vi "Check PC Time.vi"(8 "Error in":errorcluster, 11 "License File Data Out":T1) -> (0 "Error out":errorcluster, 3 "ValidTime?":bool)   [LabVIEW 2022 SP3]
uses:
  Controls/License Types.ctl
  Controls/License File Data.ctl
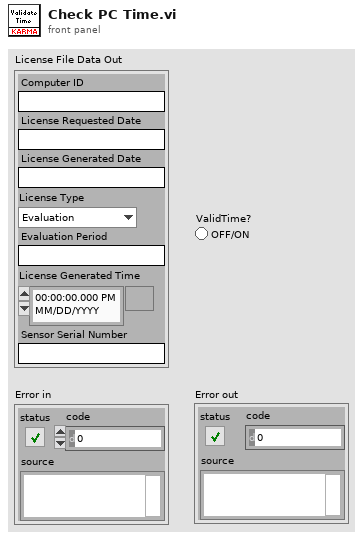
[diagram p1: front panel]
types:
  T1 = typedef "License File Data.ctl" = cluster{"Computer ID":string, "License Requested Date":string, "License Generated Date":string, "License Type":T2, "Evaluation Period":string, "License Generated Time":timestamp, "Sensor Serial Number":string}
  T2 = typedef "License Types.ctl" = enum16{"Evaluation", "Professional"}
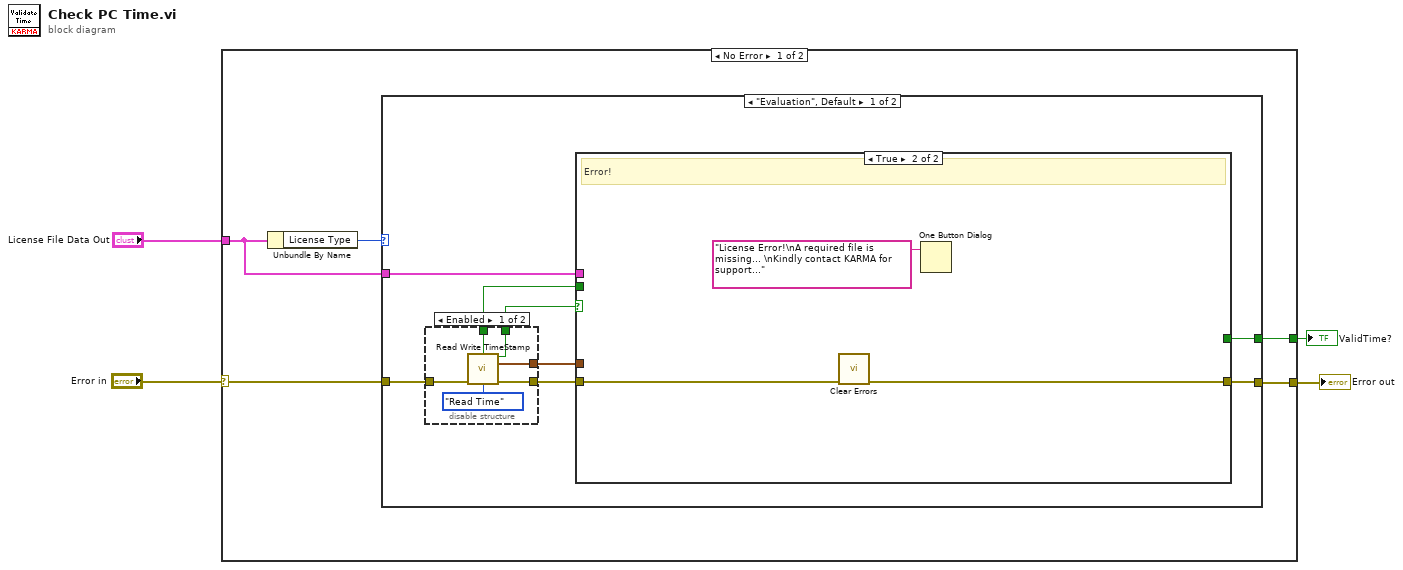
[diagram p0: block diagram]
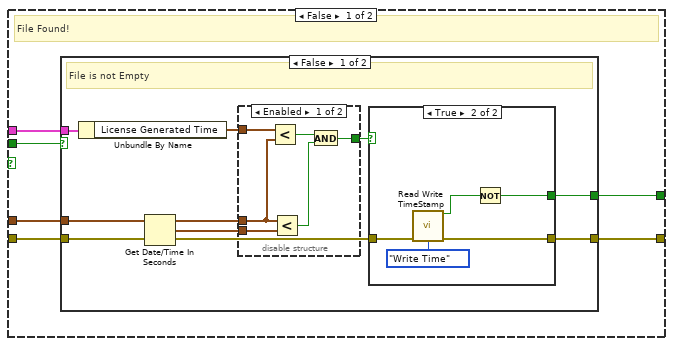
[diagram p3: hidden frame]
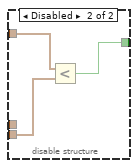
[diagram p4: hidden frame]
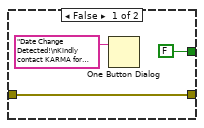
[diagram p5: hidden frame]
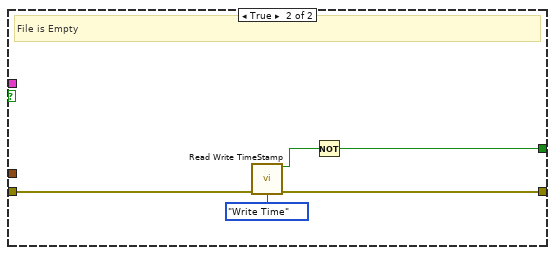
[diagram p6: hidden frame]
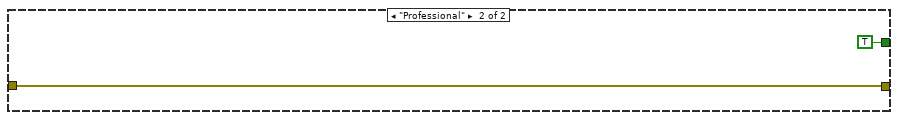
[diagram p7: hidden frame]
diagram:
  n1 = case shown="No Error" "Error in" {
    selector: "Error in" -> [w6 w65]
    tunnel: "License File Data Out" -> [w8 _]
    tunnel: [w7 w65] -> w3
    tunnel: [w5 _] -> w1
    frame No Error {
      n2 = Unbundle By Name(w8) -> ("License Type"=w9:T2)
      n3 = case shown="\"Evaluation\", Default" w9 {
        tunnel: w8 -> [w13 _]
        tunnel: w6 -> [w17 w64]
        tunnel: [w15 w64] -> w7
        tunnel: [w11 TRUE] -> w5
        frame "Evaluation", Default {
          n4 = disable-structure shown="Enabled" {
            disable-tunnel: w17 -> [w22 _]
            disable-tunnel: [w21 _] -> w16
            disable-tunnel: [w20 _] -> w14
            disable-tunnel: [w19 _] -> w12
            disable-tunnel: [w18 _] -> w10
            frame Enabled {
              n5 = call "Read Write TimeStamp.vi"("Error in"=w22, "Enum"=enum16{"Read Time", "Write Time"}."Read Time") -> ("isEmpty?"=w18:bool, "Error?"=w19:bool, "Time Stamp"=w20:timestamp, "Error out"=w21:errorcluster)  [unwired: 10 in]
            }
            frame Disabled {
            }
          }
          n6 = case shown="True" w12 {
            tunnel: w16 -> [w28 w62]
            tunnel: [w27 w60] -> w15
            tunnel: w14 -> [w25 _]
            tunnel: w13 -> [w29 _]
            tunnel: [w26 _] -> w11
            tunnel: w10 -> [w24 _]
            frame False {
              # "File Found!"
              n7 = case shown="False" w24 {
                tunnel: w29 -> [w37 _]
                tunnel: w28 -> [w35 w57]
                tunnel: [w34 w56] -> w27
                tunnel: [w33 w55] -> w26
                tunnel: w25 -> [w32 _]
                frame False {
                  # "File is not Empty"
                  n8 = Unbundle By Name(w37) -> ("License Generated Time"=w36:timestamp)
                  n9 = Get Date/Time In Seconds() -> (seconds since 1Jan1904=w31:timestamp)
                  n10 = disable-structure shown="Enabled" {
                    disable-tunnel: w36 -> [w43 w46]
                    disable-tunnel: w32 -> [w38 _]
                    disable-tunnel: w31 -> [w42 w45]
                    disable-tunnel: [w39 w44] -> w30
                    frame Enabled {
                      n11 = Less?(x=w43, y=w38) -> (x < y?=w41:bool)
                      n12 = Less?(x=w38, y=w42) -> (x < y?=w40:bool)
                      n13 = And(x=w41, y=w40) -> (x .and. y?=w39:bool)
                    }
                    frame Disabled {
                      n14 = Less?(x=w46, y=w45) -> (x < y?=w44:bool)
                    }
                  }
                  n15 = case shown="True" w30 {
                    tunnel: w35 -> [w48 w53]
                    tunnel: [w48 w52] -> w34
                    tunnel: [FALSE w50] -> w33
                    frame False {
                      n16 = One Button Dialog(message="Date Change Detected!\nKindly contact KARMA for support...") -> ()  [unwired: 1 in, 1 out]
                    }
                    frame True {
                      n17 = call "Read Write TimeStamp.vi"("Error in"=w53, "Enum"=enum16{"Read Time", "Write Time"}."Write Time") -> ("Error?"=w51:bool, "Error out"=w52:errorcluster)  [unwired: 10 in, 2 out]
                      n18 = Not(x=w51) -> (.not. x?=w50:bool)
                    }
                  }
                }
                frame True {
                  # "File is Empty"
                  n19 = call "Read Write TimeStamp.vi"("Error in"=w57, "Enum"=enum16{"Read Time", "Write Time"}."Write Time") -> ("Error?"=w59:bool, "Error out"=w56:errorcluster)  [unwired: 10 in, 2 out]
                  n20 = Not(x=w59) -> (.not. x?=w55:bool)
                }
              }
            }
            frame True {
              # "Error!"
              n21 = call <vilib>:"Clear Errors.vi"("error in (no error)"=w62) -> ("error out"=w60:errorcluster)  [unwired: 5 in, 1 out]
              n22 = One Button Dialog(message="License Error!\nA required file is missing... \nKindly contact KARMA for support...") -> ()  [unwired: 1 in, 1 out]
            }
          }
        }
        frame "Professional" {
        }
      }
    }
    frame Error {
    }
  }
  "Error out" <- w3
  "ValidTime?" <- w1
